vi "Login Rmb User.vi"(8 "error in (no error)":errorcluster, 10 "rmb user":bool, 11 "[P] User in":refnum<class "[P] User.lvclass">) -> (0 "error out":errorcluster, 3 "[P] User out":refnum<class "[P] User.lvclass">)   [LabVIEW 2020, in "[P] User.lvlib" / "[P] User.lvclass"]
uses:
  [P] User.lvclass
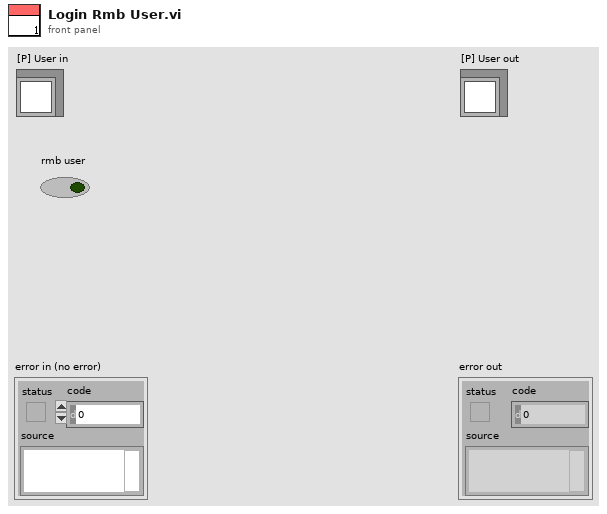
[diagram p1: front panel]
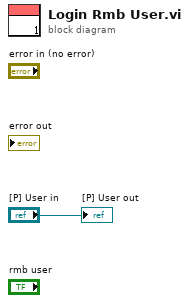
[diagram p0: block diagram]
diagram:
  "[P] User out" <- "[P] User in"
